vi "lib Parse Util.vi"() -> ()   [LabVIEW 2016]
panel:
  in  "String 5":string
  in  "Table":string[][](table)
  in  "ch numbers 2":i32[](array[numeric])=[16, 17, 18, 19, 20, 21, 22, 23, 24, 25, 26, 27, 28, 29, 30, 32, 34, 36, 37, 47, 48, 49, 50, 51, 52, 53, 54, 55, 56, 57, 58, 59, 60, 61, 62, 63, 64, 65, 66, 67, 68, 69, 70, 71, 72, 73, 74, 75, 76, 77, 78, 79, 80, 81, 82, 83, 84, 85, 86, 87, 88, 89, 90, 91, 92, 93, 94, 95, 96, 97, 98, 99, 100, 101, 102, 103, 104, 105, 106, 107, 108, 109, 110, 111, 112, 113, 114, 115, 0, 0, 0]
  in  "ch names 2":string[](array[string])=["OS_FIL1_VCTL", "OS_FIL1_ECTL", "OS_FS1_VCTL", "OS_FIL2_VCTL", "OS_FIL2_ECTL", "OS_FS2_VCTL", "CS_FIL1_VCTL", "CS_FIL1_ECTL", "CS_FS1_VCTL", "CS_FIL2_VCTL", "CS_FIL2_ECTL", "CS_FS2_VCTL", "DT1_VCTL", "DT2_VCTL", "QB_VCTL", "FIL_ON_CTRL", "ROD_AC", "ROD_DC", "RF_FREQ", "FIL_SEL", "BA_FIL_VCTL", "CS_NZ_VCTL", "MT_MU1_VCTL", "MT_MU2_VCTL", "CS_EA1_VCTL", "CS_AN1_VCTL", "CS_EA2_VCTL", "CS_AN2_VCTL", "QD_BS_VCTL", "MT_EZ_VCTL", "MT_MA1_VCTL", "MT_MA2_VCTL", "MT_WD_VCTL", "MT_FC_VCTL", "OS_EA1_VCTL", "OS_RES1_VCTL", "OS_EA2_VCTL", "OS_RES2_VCTL", "OS_OL1_VCTL", "OS_OL2_VCTL", "OS_COLA_VCTL", "OS_COLB_VCTL", "CS_IA_VCTL", "CS_RP_VCTL", "CS_RS_VCTL", "DAC8B_SPARE1", "DAC8B_SPARE2", "DAC8B_SPARE3", "IA_L1_VCTL", "IA_L2_VCTL", "IA_L4A_VCTL", "IA_L4B_VCTL", "IA_L5_VCTL", "IA_L6_VCTL", "OS_EF1A_VCTL", "OS_EF1B_VCTL", "OS_EF1C_VCTL", "OS_EF1D_VCTL", "OS_EF2A_VCTL", "OS_EF2B_VCTL", "OS_EF2C_VCTL", "OS_EF2D_VCTL", "CS_EF1A_VCTL", "CS_EF1B_VCTL", "CS_EF1C_VCTL", "CS_EF1D_VCTL", "CS_EF2A_VCTL", "CS_EF2B_VCTL", "CS_EF2C_VCTL", "CS_EF2D_VCTL", "DAC12USPARE1", "DAC12USPARE2", "OS_OL4_VCTL", "CS_IFA_VCTL", "CS_IFB_VCTL", "SL_TB_VCTL", "SL_BB_VCTL", "SL_BF_VCTL", "SL_EL_VCTL", "OS_OL3_VCTL", "SL_TF_VCTL", "OS_OL5_VCTL", "OS_OL6_VCTL", "DAC12BSPARE1", "DAC12BSPARE2", "DAC12BSPARE3", "DAC16BSPARE1", "DAC16BSPARE2", "", "", ""]
  out "ch numbers":i32[](array[numeric])=[16, 17, 18, 19, 20, 21, 22, 23, 24, 25, 26, 27, 28, 29, 30, 32, 34, 36, 37, 47, 48, 49, 50, 51, 52, 53, 54, 55, 56, 57, 58, 59, 60, 61, 62, 63, 64, 65, 66, 67, 68, 69, 70, 71, 72, 73, 74, 75, 76, 77, 78, 79, 80, 81, 82, 83, 84, 85, 86, 87, 88, 89, 90, 91, 92, 93, 94, 95, 96, 97, 98, 99, 100, 101, 102, 103, 104, 105, 106, 107, 108, 109, 110, 111, 112, 113, 114, 115, 0, 0, 0]
  out "ch names":string[](array[string])=["OS_FIL1_VCTL", "OS_FIL1_ECTL", "OS_FS1_VCTL", "OS_FIL2_VCTL", "OS_FIL2_ECTL", "OS_FS2_VCTL", "CS_FIL1_VCTL", "CS_FIL1_ECTL", "CS_FS1_VCTL", "CS_FIL2_VCTL", "CS_FIL2_ECTL", "CS_FS2_VCTL", "DT1_VCTL", "DT2_VCTL", "QB_VCTL", "FIL_ON_CTRL", "ROD_AC", "ROD_DC", "RF_FREQ", "FIL_SEL", "BA_FIL_VCTL", "CS_NZ_VCTL", "MT_MU1_VCTL", "MT_MU2_VCTL", "CS_EA1_VCTL", "CS_AN1_VCTL", "CS_EA2_VCTL", "CS_AN2_VCTL", "QD_BS_VCTL", "MT_EZ_VCTL", "MT_MA1_VCTL", "MT_MA2_VCTL", "MT_WD_VCTL", "MT_FC_VCTL", "OS_EA1_VCTL", "OS_RES1_VCTL", "OS_EA2_VCTL", "OS_RES2_VCTL", "OS_OL1_VCTL", "OS_OL2_VCTL", "OS_COLA_VCTL", "OS_COLB_VCTL", "CS_IA_VCTL", "CS_RP_VCTL", "CS_RS_VCTL", "DAC8B_SPARE1", "DAC8B_SPARE2", "DAC8B_SPARE3", "IA_L1_VCTL", "IA_L2_VCTL", "IA_L4A_VCTL", "IA_L4B_VCTL", "IA_L5_VCTL", "IA_L6_VCTL", "OS_EF1A_VCTL", "OS_EF1B_VCTL", "OS_EF1C_VCTL", "OS_EF1D_VCTL", "OS_EF2A_VCTL", "OS_EF2B_VCTL", "OS_EF2C_VCTL", "OS_EF2D_VCTL", "CS_EF1A_VCTL", "CS_EF1B_VCTL", "CS_EF1C_VCTL", "CS_EF1D_VCTL", "CS_EF2A_VCTL", "CS_EF2B_VCTL", "CS_EF2C_VCTL", "CS_EF2D_VCTL", "DAC12USPARE1", "DAC12USPARE2", "OS_OL4_VCTL", "CS_IFA_VCTL", "CS_IFB_VCTL", "SL_TB_VCTL", "SL_BB_VCTL", "SL_BF_VCTL", "SL_EL_VCTL", "OS_OL3_VCTL", "SL_TF_VCTL", "OS_OL5_VCTL", "OS_OL6_VCTL", "DAC12BSPARE1", "DAC12BSPARE2", "DAC12BSPARE3", "DAC16BSPARE1", "DAC16BSPARE2", "", "", ""]
  in  "String 4":string="OS_FIL1_VCTL  = 16\nOS_FIL1_ECTL  = 17\nOS_FS1_VCTL   = 18\nOS_FIL2_VCTL  = 19\nOS_FIL2_ECTL  = 20\nOS_FS2_VCTL   = 21\nCS_FIL1_VCTL  = 22\nCS_FIL1_ECTL  = 23\nCS_FS1_VCTL   = 24\nCS_FIL2_VCTL  = 25\nCS_FIL2_ECTL  = 26\nCS_FS2_VCTL   = 27\nDT1_VCTL      = 28\nDT2_VCTL      = 29\nQB_VCTL       = 30\nFIL_ON_CTRL   = 32\nROD_AC        = 34\nROD_DC        = 36\nRF_FREQ       = 37\nFIL_SEL       = 47\nBA_FIL_VCTL   = 48\nCS_NZ_VCTL    = 49\nMT_MU1_VCTL   = 50\nMT_MU2_VCTL   = 51\nCS_EA1_VCTL   = 52\nCS_AN1_VCTL   = 53\nCS_EA2_VCTL   = 54\nCS_AN2_VCTL   = 55\nQD_BS_VCTL    = 56\nMT_EZ_VCTL    = 57\nMT_MA1_VCTL   = 58\nMT_MA2_VCTL   = 59\nMT_WD_VCTL    = 60\nMT_FC_VCTL    = 61\nOS_EA1_VCTL   = 62\nOS_RES1_VCTL  = 63\nOS_EA2_VCTL   = 64\nOS_RES2_VCTL  = 65\nOS_OL1_VCTL   = 66\nOS_OL2_VCTL   = 67\nOS_COLA_VCTL  = 68\nOS_COLB_VCTL  = 69\nCS_IA_VCTL    = 70\nCS_RP_VCTL    = 71\nCS_RS_VCTL    = 72\nDAC8B_SPARE1  = 73\nDAC8B_SPARE2  = 74\nDAC8B_SPARE3  = 75\nIA_L1_VCTL    = 76\nIA_L2_VCTL    = 77\nIA_L4A_VCTL   = 78\nIA_L4B_VCTL   = 79\nIA_L5_VCTL    = 80\nIA_L6_VCTL    = 81\nOS_EF1A_VCTL  = 82\nOS_EF1B_VCTL  = 83\nOS_EF1C_VCTL  = 84\nOS_EF1D_VCTL  = 85\nOS_EF2A_VCTL  = 86\nOS_EF2B_VCTL  = 87\nOS_EF2C_VCTL  = 88\nOS_EF2D_VCTL  = 89\nCS_EF1A_VCTL  = 90\nCS_EF1B_VCTL  = 91\nCS_EF1C_VCTL  = 92\nCS_EF1D_VCTL  = 93\nCS_EF2A_VCTL  = 94\nCS_EF2B_VCTL  = 95\nCS_EF2C_VCTL  = 96\nCS_EF2D_VCTL  = 97\nDAC12USPARE1  = 98\nDAC12USPARE2  = 99\nOS_OL4_VCTL   = 100\nCS_IFA_VCTL   = 101\nCS_IFB_VCTL   = 102\nSL_TB_VCTL    = 103\nSL_BB_VCTL    = 104\nSL_BF_VCTL    = 105\nSL_EL_VCTL    = 106\nOS_OL3_VCTL   = 107\nSL_TF_VCTL    = 108\nOS_OL5_VCTL   = 109\nOS_OL6_VCTL   = 110\nDAC12BSPARE1  = 111\nDAC12BSPARE2  = 112\nDAC12BSPARE3  = 113\nDAC16BSPARE1  = 114\nDAC16BSPARE2  = 115\n"
  in  "String 3":string="data \"OS_FS1_VCTL\",     0.0,        0.0,        2\ndata \"OS_EF1A_VCTL\",    0.0,        0.0,        2\ndata \"OS_EF1B_VCTL\",    0.0,        0.0,        2\ndata \"OS_EF1C_VCTL\",\t0.0,\t\t0.0,\t\t2\ndata \"OS_EF1D_VCTL\",\t0.0,\t\t0.0,\t\t2\ndata \"OS_EA1_VCTL\",\t    0.0,\t\t0.0,\t\t2\ndata \"OS_RES1_VCTL\",\t0.0,\t\t0.0,\t\t2\ndata \"OS_FS2_VCTL\",\t    0.0,\t\t0.0,\t\t2\ndata \"OS_EF2A_VCTL\",\t0.0,\t\t0.0,\t\t2\ndata \"OS_EF2B_VCTL\",\t0.0,\t\t0.0,\t\t2\ndata \"OS_EF2C_VCTL\",\t0.0,\t\t0.0,\t\t2\ndata \"OS_EF2D_VCTL\",\t0.0,\t\t0.0,\t\t2\ndata \"OS_EA2_VCTL\",\t    0.0,\t\t0.0,\t\t2\ndata \"OS_RES2_VCTL\",\t0.0,\t\t0.0,\t\t2\ndata \"OS_COLA_VCTL\",\t0.0,\t\t0.0,\t\t2\ndata \"OS_COLB_VCTL\",\t0.0,\t\t0.0,\t\t2\ndata \"OS_OL1_VCTL\",\t    0.0,\t\t0.0,\t\t2\ndata \"OS_OL2_VCTL\",\t    0.0,\t\t0.0,\t\t2\ndata \"OS_OL3_VCTL\",\t    0.0,\t\t0.0,\t\t2\ndata \"OS_OL4_VCTL\",\t    0.0,\t\t0.0,\t\t2\ndata \"OS_OL5_VCTL\",\t    0.0,\t\t0.0,\t\t2\ndata \"OS_OL6_VCTL\",\t    0.0,\t\t0.0,\t\t2\ndata \"CS_FS1_VCTL\",\t    0.0,\t\t0.0,\t\t2\ndata \"CS_EF1A_VCTL\",\t0.0,\t\t0.0,\t\t1\ndata \"CS_EF1B_VCTL\",\t0.0,\t\t0.0,\t\t1\ndata \"CS_EF1C_VCTL\",\t0.0,\t\t0.0,\t\t1\ndata \"CS_EF1D_VCTL\",\t0.0,\t\t0.0,\t\t1\ndata \"CS_EA1_VCTL\",\t    0.0,\t\t0.0,\t\t1\ndata \"CS_AN1_VCTL\",\t    0.0,\t\t0.0,\t\t1\ndata \"CS_FS2_VCTL\",\t    0.0,\t\t0.0,\t\t1\ndata \"CS_EF2A_VCTL\",\t0.0,\t\t0.0,\t\t1\ndata \"CS_EF2B_VCTL\",\t0.0,\t\t0.0,\t\t1\ndata \"CS_EF2C_VCTL\",\t0.0,\t\t0.0,\t\t1\ndata \"CS_EF2D_VCTL\",\t0.0,\t\t0.0,\t\t1\ndata \"CS_EA2_VCTL\",\t    0.0,\t\t0.0,\t\t1\ndata \"CS_AN2_VCTL\",\t    0.0,\t\t0.0,\t\t1\ndata \"CS_IA_VCTL\",\t    0.0,\t\t0.0,\t\t1\ndata \"CS_IFA_VCTL\",\t    0.0,\t\t0.0,\t\t1\ndata \"CS_IFB_VCTL\",\t    0.0,\t\t0.0,\t\t1\ndata \"CS_NZ_VCTL\",\t    0.0,\t\t0.0,\t\t1\ndata \"CS_RP_VCTL\",\t    0.0,\t\t0.0,\t\t1\ndata \"CS_RS_VCTL\",\t    0.0,\t\t0.0,\t\t1\ndata \"MT_FC_VCTL\",\t    0.0,\t\t0.0,\t\t1\ndata \"QD_BS_VCTL\",\t    0.0,\t\t0.0,\t\t1\ndata \"MT_MA1_VCTL\",\t    0.0,\t\t0.0,\t\t1\ndata \"MT_MA2_VCTL\",\t    0.0,\t\t0.0,\t\t1\ndata \"MT_EZ_VCTL\",\t    0.0,\t\t0.0,\t\t1\ndata \"MT_WD_VCTL\",\t    0.0,\t\t0.0,\t\t1\ndata \"SL_BB_VCTL\",\t    0.0,\t\t0.0,\t\t1\ndata \"SL_TF_VCTL\",\t    0.0,\t\t0.0,\t\t1\ndata \"SL_BF_VCTL\",\t    0.0,\t\t0.0,\t\t1\ndata \"SL_TB_VCTL\",\t    0.0,\t\t0.0,\t\t1\ndata \"SL_EL_VCTL\",\t    0.0,\t\t0.0,\t\t1\ndata \"IA_L1_VCTL\",\t    0.0,\t\t0.0,\t\t1\ndata \"IA_L2_VCTL\",\t    0.0,\t\t0.0,\t\t1\ndata \"IA_L4A_VCTL\",\t    0.0,\t\t0.0,\t\t1\ndata \"IA_L4B_VCTL\",\t    0.0,\t\t0.0,\t\t1\ndata \"IA_L5_VCTL\",\t    0.0,\t\t0.0,\t\t1\ndata \"IA_L6_VCTL\",\t    0.0,\t\t0.0,\t\t1\n"
  out "concatenated string":string
  in  "line number base":i32
  out "Array":string[](array[string])
  out "String 2":string
  out "Array 2":string[](array[string])
  in  "String":string="data OS_FS1_VCTL,\t\"OS_FS1_VCTL\",\t -20,\t0.0,\t0.0,\t0.0,\t0.0,\t0\ndata OS_EF1A_VCTL,\t\"OS_EF1A_VCTL\",\t -20,\t0.0,\t0.0,\t0.0,\t0.0,\t0\ndata OS_EF1B_VCTL,\t\"OS_EF1B_VCTL\",\t -20,\t0.0,\t0.0,\t0.0,\t0.0,\t0\ndata OS_EF1C_VCTL,\t\"OS_EF1C_VCTL\",\t -20,\t0.0,\t0.0,\t0.0,\t0.0,\t0\ndata OS_EF1D_VCTL,\t\"OS_EF1D_VCTL\",\t -20,\t0.0,\t0.0,\t0.0,\t0.0,\t0\ndata OS_EA1_VCTL,\t\"OS_EA1_VCTL\",\t 50,\t0.0,\t0.0,\t0.0,\t0.0,\t0\ndata OS_RES1_VCTL,\t\"OS_RES1_VCTL\",\t 50,\t0.0,\t0.0,\t0.0,\t0.0,\t0\ndata OS_FS2_VCTL,\t\"OS_FS2_VCTL\",\t -20,\t0.0,\t0.0,\t0.0,\t0.0,\t0\ndata OS_EF2A_VCTL,\t\"OS_EF2A_VCTL\",\t -20,\t0.0,\t0.0,\t0.0,\t0.0,\t0\ndata OS_EF2B_VCTL,\t\"OS_EF2B_VCTL\",\t -20,\t0.0,\t0.0,\t0.0,\t0.0,\t0\ndata OS_EF2C_VCTL,\t\"OS_EF2C_VCTL\",\t -20,\t0.0,\t0.0,\t0.0,\t0.0,\t0\ndata OS_EF2D_VCTL,\t\"OS_EF2D_VCTL\",\t -20,\t0.0,\t0.0,\t0.0,\t0.0,\t0\ndata OS_EA2_VCTL,\t\"OS_EA2_VCTL\",\t -20,\t0.0,\t0.0,\t0.0,\t0.0,\t0\ndata OS_RES2_VCTL,\t\"OS_RES2_VCTL\",\t -30,\t0.0,\t0.0,\t0.0,\t0.0,\t0\ndata OS_COLA_VCTL,\t\"OS_COLA_VCTL\",\t -30,\t0.0,\t0.0,\t0.0,\t0.0,\t0\ndata OS_COLB_VCTL,\t\"OS_COLB_VCTL\",\t -30,\t0.0,\t0.0,\t0.0,\t0.0,\t0\ndata OS_OL1_VCTL,\t\"OS_OL1_VCTL\",\t -5,\t0.0,\t0.0,\t0.0,\t0.0,\t0\ndata OS_OL2_VCTL,\t\"OS_OL2_VCTL\",\t -5,\t0.0,\t0.0,\t0.0,\t0.0,\t0\ndata OS_OL3_VCTL,\t\"OS_OL3_VCTL\",\t -30,\t0.0,\t0.0,\t0.0,\t0.0,\t0\ndata OS_OL4_VCTL,\t\"OS_OL4_VCTL\",\t -50,\t0.0,\t0.0,\t0.0,\t0.0,\t0\ndata OS_OL5_VCTL,\t\"OS_OL5_VCTL\",\t -100,\t0.0,\t0.0,\t0.0,\t0.0,\t0\ndata OS_OL6_VCTL,\t\"OS_OL6_VCTL\",\t -100,\t0.0,\t0.0,\t0.0,\t0.0,\t0\ndata CS_FS1_VCTL,\t\"CS_FS1_VCTL\",\t -20,\t0.0,\t0.0,\t0.0,\t0.0,\t0\ndata CS_EF1A_VCTL,\t\"CS_EF1A_VCTL\",\t -20,\t0.0,\t0.0,\t0.0,\t0.0,\t0\ndata CS_EF1B_VCTL,\t\"CS_EF1B_VCTL\",\t -20,\t0.0,\t0.0,\t0.0,\t0.0,\t0\ndata CS_EF1C_VCTL,\t\"CS_EF1C_VCTL\",\t -20,\t0.0,\t0.0,\t0.0,\t0.0,\t0\ndata CS_EF1D_VCTL,\t\"CS_EF1D_VCTL\",\t -20,\t0.0,\t0.0,\t0.0,\t0.0,\t0\ndata CS_EA1_VCTL,\t\"CS_EA1_VCTL\",\t 50,\t0.0,\t0.0,\t0.0,\t0.0,\t0\ndata CS_AN1_VCTL,\t\"CS_AN1_VCTL\",\t 50,\t0.0,\t0.0,\t0.0,\t0.0,\t0\ndata CS_FS2_VCTL,\t\"CS_FS2_VCTL\",\t -20,\t0.0,\t0.0,\t0.0,\t0.0,\t0\ndata CS_EF2A_VCTL,\t\"CS_EF2A_VCTL\",\t -20,\t0.0,\t0.0,\t0.0,\t0.0,\t0\ndata CS_EF2B_VCTL,\t\"CS_EF2B_VCTL\",\t -20,\t0.0,\t0.0,\t0.0,\t0.0,\t0\ndata CS_EF2C_VCTL,\t\"CS_EF2C_VCTL\",\t -20,\t0.0,\t0.0,\t0.0,\t0.0,\t0\ndata CS_EF2D_VCTL,\t\"CS_EF2D_VCTL\",\t -20,\t0.0,\t0.0,\t0.0,\t0.0,\t0\ndata CS_EA2_VCTL,\t\"CS_EA2_VCTL\",\t 50,\t0.0,\t0.0,\t0.0,\t0.0,\t0\ndata CS_AN2_VCTL,\t\"CS_AN2_VCTL\",\t 50,\t0.0,\t0.0,\t0.0,\t0.0,\t0\ndata CS_IA_VCTL,\t\"CS_IA_VCTL\",\t 5.0,\t0.0,\t0.0,\t0.0,\t0.0,\t0\ndata CS_IFA_VCTL,\t\"CS_IFA_VCTL\",\t -50,\t0.0,\t0.0,\t0.0,\t0.0,\t0\ndata CS_IFB_VCTL,\t\"CS_IFB_VCTL\",\t -50,\t0.0,\t0.0,\t0.0,\t0.0,\t0\ndata CS_NZ_VCTL,\t\"CS_NZ_VCTL\",\t -50,\t0.0,\t0.0,\t0.0,\t0.0,\t0\ndata CS_RP_VCTL,\t\"CS_RP_VCTL\",\t -5,\t0.0,\t0.0,\t0.0,\t0.0,\t0\ndata CS_RS_VCTL,\t\"CS_RS_VCTL\",\t -5,\t0.0,\t0.0,\t0.0,\t0.0,\t0\ndata MT_FC_VCTL,\t\"MT_FC_VCTL\",\t -30,\t0.0,\t0.0,\t0.0,\t0.0,\t0\ndata QD_BS_VCTL,\t\"QD_BS_VCTL\",\t -30,\t0.0,\t0.0,\t0.0,\t0.0,\t0\ndata MT_MA1_VCTL,\t\"MT_MA1_VCTL\",\t -40,\t0.0,\t0.0,\t0.0,\t0.0,\t0\ndata MT_MA2_VCTL,\t\"MT_MA2_VCTL\",\t -40,\t0.0,\t0.0,\t0.0,\t0.0,\t0\ndata MT_EZ_VCTL,\t\"MT_EZ_VCTL\",\t -40,\t0.0,\t0.0,\t0.0,\t0.0,\t0\ndata MT_WD_VCTL,\t\"MT_WD_VCTL\",\t -40,\t0.0,\t0.0,\t0.0,\t0.0,\t0\ndata SL_BB_VCTL,\t\"SL_BB_VCTL\",\t -100,\t0.0,\t0.0,\t0.0,\t0.0,\t0\ndata SL_TF_VCTL,\t\"SL_TF_VCTL\",\t -100,\t0.0,\t0.0,\t0.0,\t0.0,\t0\ndata SL_BF_VCTL,\t\"SL_BF_VCTL\",\t -100,\t0.0,\t0.0,\t0.0,\t0.0,\t0\ndata SL_TB_VCTL,\t\"SL_TB_VCTL\",\t -100,\t0.0,\t0.0,\t0.0,\t0.0,\t0\ndata SL_EL_VCTL,\t\"SL_EL_VCTL\",\t 100,\t0.0,\t0.0,\t0.0,\t0.0,\t0\ndata IA_L1_VCTL,\t\"IA_L1_VCTL\",\t -100,\t0.0,\t0.0,\t0.0,\t0.0,\t0\ndata IA_L2_VCTL,\t\"IA_L2_VCTL\",\t -100,\t0.0,\t0.0,\t0.0,\t0.0,\t0\ndata IA_L4A_VCTL,\t\"IA_L4A_VCTL\",\t -50,\t0.0,\t0.0,\t0.0,\t0.0,\t0\ndata IA_L4B_VCTL,\t\"IA_L4B_VCTL\",\t -50,\t0.0,\t0.0,\t0.0,\t0.0,\t0\ndata IA_L5_VCTL,\t\"IA_L5_VCTL\",\t -100,\t0.0,\t0.0,\t0.0,\t0.0,\t0\ndata IA_L6_VCTL,\t\"IA_L6_VCTL\",\t -100,\t0.0,\t0.0,\t0.0,\t0.0,\t0\n"
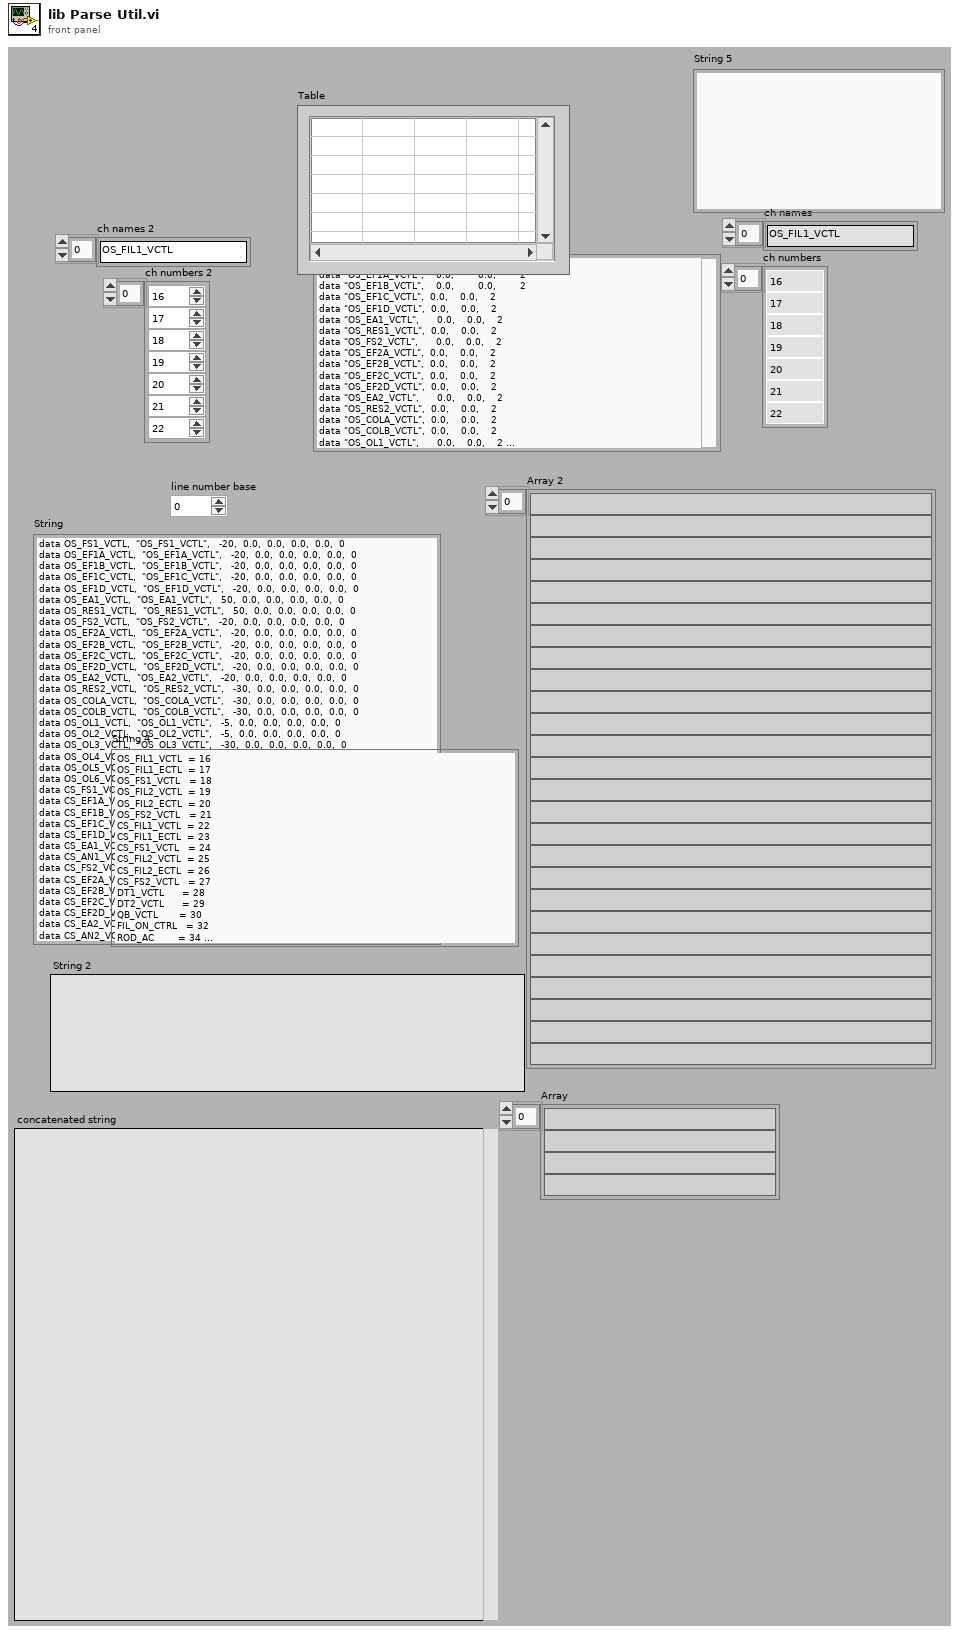
[diagram p1: front panel]
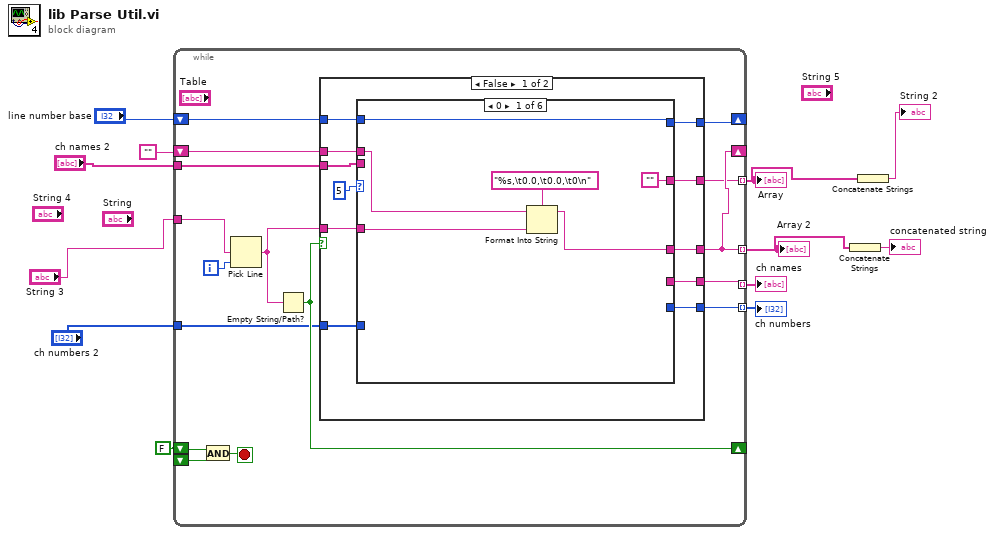
[diagram p0: block diagram]
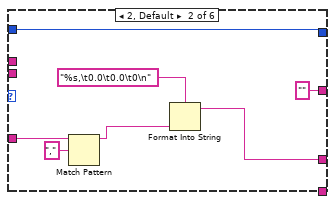
[diagram p2: hidden frame]
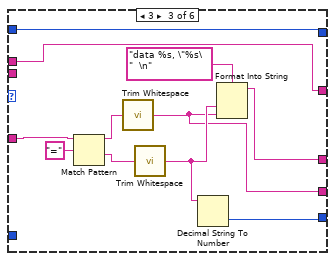
[diagram p3: hidden frame]
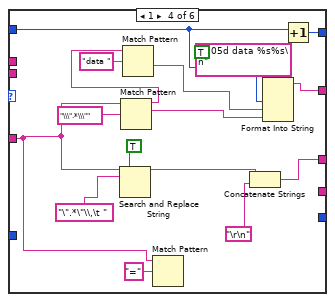
[diagram p4: hidden frame]
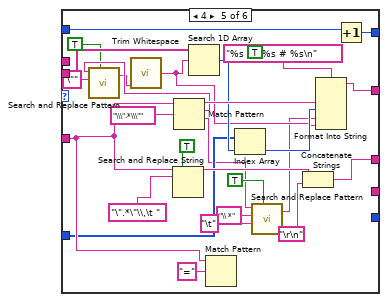
[diagram p5: hidden frame]
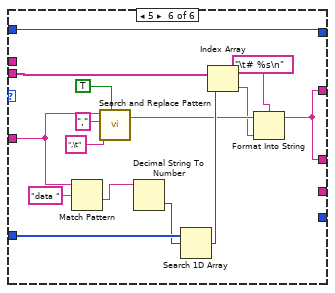
[diagram p6: hidden frame]
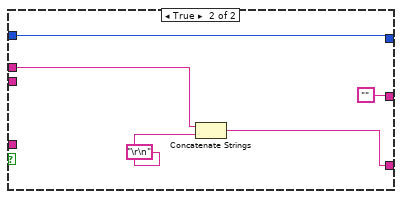
[diagram p7: hidden frame]
diagram:
  w11 = FALSE
  n1 = while {
    tunnel: "String 3" -> [w28]
    tunnel: [w24] -> w7 mode=indexing
    shift-right: [w24] -> _
    shift-left: "" -> [w25]
    shift-right: [w20] -> _
    shift-left: w11 -> [w22]
    shift-left: w11 -> [w21]
    tunnel: [w19] -> w9 mode=indexing
    shift-right: [w17] -> _
    shift-left: "line number base" -> [w18]
    tunnel: [w16] -> w5 mode=indexing
    tunnel: [w15] -> w4 mode=indexing
    tunnel: "ch names 2" -> [w14]
    tunnel: "ch numbers 2" -> [w13]
    i -> [w27]
    stop <- w23 stop-if-true
    n2 = And(x=w22, y=w21) -> (x .and. y?=w23:bool)
    n3 = Pick Line(multi-line string=w28, line index=w27) -> (output string=w26:string)  [unwired: 1 in]
    n4 = Empty String/Path?(string/path=w26) -> (empty?=w20:bool)
    n5 = case shown="False" w20 {
      tunnel: w26 -> [w39 _]
      tunnel: w25 -> [w38 w126]
      tunnel: [w37 w124] -> w24
      tunnel: [w35 ""] -> w19
      tunnel: w18 -> [w34 w122]
      tunnel: [w33 w122] -> w17
      tunnel: [w32 _] -> w15
      tunnel: [w31 _] -> w16
      tunnel: w14 -> [w30 _]
      tunnel: w13 -> [w29 _]
      frame False {
        n6 = case shown="0" 5 {
          tunnel: w39 -> [w42 w52 w62 w67 w95 w117]
          tunnel: w38 -> [w44 _ w57 _ _ _]
          tunnel: [w43 w47 w58 w69 w97 w109] -> w37
          tunnel: ["" "" w57 w74 w101 w109] -> w35
          tunnel: w34 -> [w40 w48 w56 w72 w99 w108]
          tunnel: [w40 w48 w56 w73 w100 w108] -> w33
          tunnel: [_ _ w53 _ _ _] -> w32
          tunnel: [_ _ w54 _ _ _] -> w31
          tunnel: w30 -> [_ _ _ _ w93 w118]
          tunnel: w29 -> [_ _ _ _ w91 w120]
          frame 0 {
            n7 = Format Into String(format string="%s,\t0.0,\t0.0,\t0\n", initial string=w44, w42) -> (resulting string=w43:string)  [unwired: 1 in, 1 out]
          }
          frame 2, Default {
            n8 = Match Pattern(string=w52, regular expression=",") -> (before substring=w49:string)  [unwired: 1 in, 3 out]
            n9 = Format Into String(format string="%s,\t0.0\t0.0\t0\n", w49) -> (resulting string=w47:string)  [unwired: 2 in, 1 out]
          }
          frame 3 {
            n10 = Match Pattern(string=w62, regular expression="=") -> (before substring=w61:string, after substring=w59:string)  [unwired: 1 in, 2 out]
            n11 = call <vilib>:"Trim Whitespace.vi"("string"=w61) -> ("trimmed string"=w54:string)  [unwired: 1 in]
            n12 = call <vilib>:"Trim Whitespace.vi"("string"=w59) -> ("trimmed string"=w55:string)  [unwired: 1 in]
            n13 = Decimal String To Number(string=w55) -> (number=w53:i32)  [unwired: 2 in, 1 out]
            n14 = Format Into String(format string="data %s, \"%s\"  \n", w55, w54) -> (resulting string=w58:string)  [unwired: 2 in, 1 out]
          }
          frame 1 {
            (unwired) TRUE ("replace all? (F)")
            n15 = Search and Replace String(replace all?=TRUE ("replace all? (F)"), input string=w67, search string="\".*\"\\,\t " ("regular expression")) -> (result string=w76:string)  [unwired: 5 in, 3 out]
            n16 = Match Pattern(string=w67, regular expression="\\\".*\\\"") -> (before substring=w66:string, match substring=w70:string)  [unwired: 1 in, 2 out]
            n17 = Match Pattern(string=w66, regular expression="data ") -> (after substring=w64:string)  [unwired: 1 in, 3 out]
            n18 = Match Pattern(string=w67, regular expression="=") -> ()  [unwired: 1 in, 4 out]
            n19 = Concatenate Strings(w76, "\r\n") -> (w69:string)
            n20 = Format Into String(format string="%05d data %s%s\n", w72, w64, w70) -> (resulting string=w74:string)  [unwired: 2 in, 1 out]
            n21 = Increment(x=w72) -> (x+1=w73:i32)
          }
          frame 4 {
            (unwired) TRUE ("replace all? (F)")
            n22 = Search and Replace String(replace all?=TRUE ("replace all? (F)"), input string=w95, search string="\".*\"\\,\t " ("regular expression")) -> (result string=w103:string)  [unwired: 5 in, 3 out]
            n23 = Match Pattern(string=w95, regular expression="\\\".*\\\"") -> (before substring=w94:string, match substring=w89:string, after substring=w81:string)  [unwired: 1 in, 1 out]
            n24 = call <vilib>:"Search and Replace Pattern.vi"("string"=w89, "regular expression (\"\")"="\"" ("regular expression (\"\")"), "replace all? (F)"=TRUE) -> ("result string"=w86:string)  [unwired: 2 in, 1 out]
            n25 = call <vilib>:"Trim Whitespace.vi"("string"=w86) -> ("trimmed string"=w85:string)  [unwired: 1 in]
            n26 = Search 1D Array(1D array=w93, element=w85) -> (index of element=w92:i32)  [unwired: 1 in]
            n27 = Match Pattern(string=w95, regular expression="=") -> ()  [unwired: 1 in, 4 out]
            n28 = Index Array(array=w91, index=w92) -> (element=w90:i32)
            n29 = call <vilib>:"Search and Replace Pattern.vi"("string"=w81, "regular expression (\"\")"="\\ *" ("regular expression (\"\")"), "replace string (\"\")"="\t" ("replace string (\"\")"), "replace all? (F)"=TRUE) -> ("result string"=w80:string)  [unwired: 1 in, 1 out]
            n30 = Concatenate Strings(w103, "\r\n") -> (w97:string)
            n31 = Format Into String(format string="%s %d%s # %s\n", w94, w90, w80, w85) -> (resulting string=w101:string)  [unwired: 2 in, 1 out]
            n32 = Increment(x=w99) -> (x+1=w100:i32)
          }
          frame 5 {
            n33 = Match Pattern(string=w117, regular expression="data ") -> (after substring=w107:string)  [unwired: 1 in, 3 out]
            n34 = call <vilib>:"Search and Replace Pattern.vi"("string"=w117, "regular expression (\"\")"="," ("regular expression (\"\")"), "replace string (\"\")"=",\t" ("replace string (\"\")"), "replace all? (F)"=TRUE) -> ("result string"=w111:string)  [unwired: 1 in, 1 out]
            n35 = Decimal String To Number(string=w107) -> (number=w119:i32)  [unwired: 2 in, 1 out]
            n36 = Search 1D Array(1D array=w120, element=w119) -> (index of element=w113:i32)  [unwired: 1 in]
            n37 = Index Array(array=w118, index=w113) -> (element=w110:string)
            n38 = Format Into String(format string="\t# %s\n", initial string=w111, w110) -> (resulting string=w109:string)  [unwired: 1 in, 1 out]
          }
        }
      }
      frame True {
        n39 = Concatenate Strings(w126, "\r\n") -> (w124:string)
      }
    }
  }
  "Array 2" <- w7
  "Array" <- w9
  "ch names" <- w5
  "ch numbers" <- w4
  n40 = Concatenate Strings(w7) -> (→"concatenated string":string)
  n41 = Concatenate Strings(w9) -> (→"String 2":string)
